vi "Read only temperature.vi"() -> ()   [LabVIEW 2013]
doc: "This example shows how to configure a measurement and take a reading."
uses:
  <vilib>/Utility/file.llb/Read From Spreadsheet File (DBL).vi
  <instrlib>/Keithley 24XX/Public/Data/Read (Single Point).vi
  <instrlib>/Keithley 24XX/Keithley 24XX.lvlib
  <vilib>/gmath/NI_Gmath.lvlib
panel:
  in  "测量间隔（毫秒）":dbl
  out "温度-时间":dbl(graph)
  out "Temperature":dbl
  in  "定标文件":string(combo)="original.txt"
  in  "Source Mode  (0: Voltage)":u16(ring) items=["Voltage", "Current"]
  in  "Compliance  Level (0.1)":dbl=0.0001
  in  "Output Level (0)":dbl=0.002
  in  "Enable Resistance Auto Range (T:Enable)":bool=TRUE
  in  "Enable Current Auto Range (T:Enable)":bool=TRUE
  in  "Enable Voltage Auto Range (T:Enable)":bool=TRUE
  in  "Resistance Manual Range (1.0)":dbl=1.0
  in  "Current Manual Range (1.0)":dbl=1.0
  in  "Voltage Manual Range (1.0)":dbl=1.0
  out "Resistance":sgl
  out "Current":sgl
  out "Voltage":sgl
  in  "Serial Configuration":T1={"Baud Rate"=9600, "Parity"=0, "Data Bits"=8, "Stop Bits"=10, "Flow Control"=0} {"Flow Control" items=["None", "XON/XOFF", "RTS/CTS", "XON/XOFF & RTS/CTS", "DTR/DSR", "XON/XOFF & DTR/DSR"]; "Stop Bits" items=["1.0"=10, "1.5"=15, "2.0"=20]; "Data Bits" items=["7"=7, "8"=8]; "Parity" items=["None", "Odd", "Even", "Mark", "Space"]; "Baud Rate" items=["300"=300, "600"=600, "1200"=1200, "2400"=2400, "4800"=4800, "9600"=9600, "19200"=19200]}
  in  "Keithley 2400\nVISA resource name":refnum<visa-resource-name>
  # "温度测量（适用于Keithley 2400） 版本：1.1"
  # "Voltage Range Settings"
  # "Current Range Settings"
  # "Resistance Range Settings"
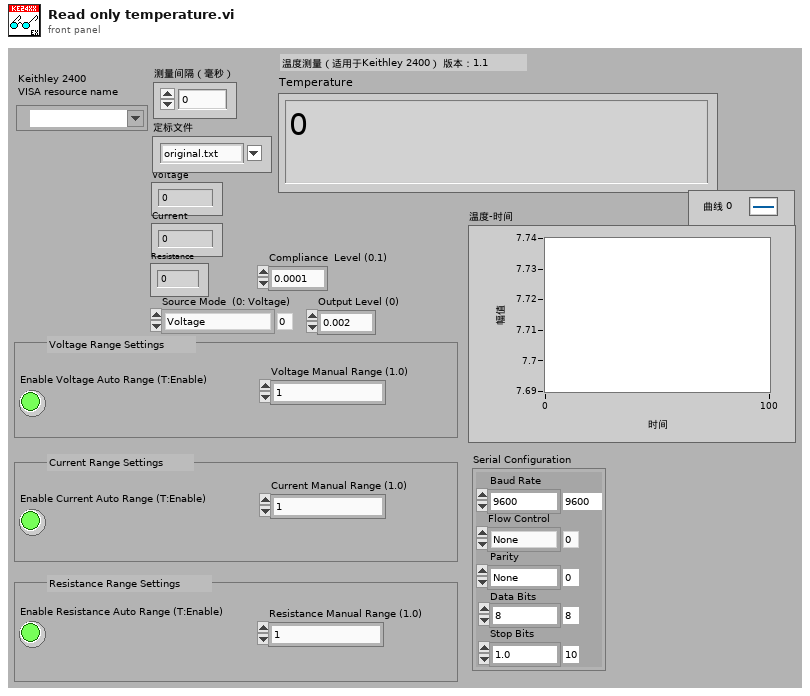
[diagram p1: front panel]
types:
  T1 = cluster{"Baud Rate":u32, "Parity":u16, "Data Bits":u16, "Stop Bits":u16, "Flow Control":u16}
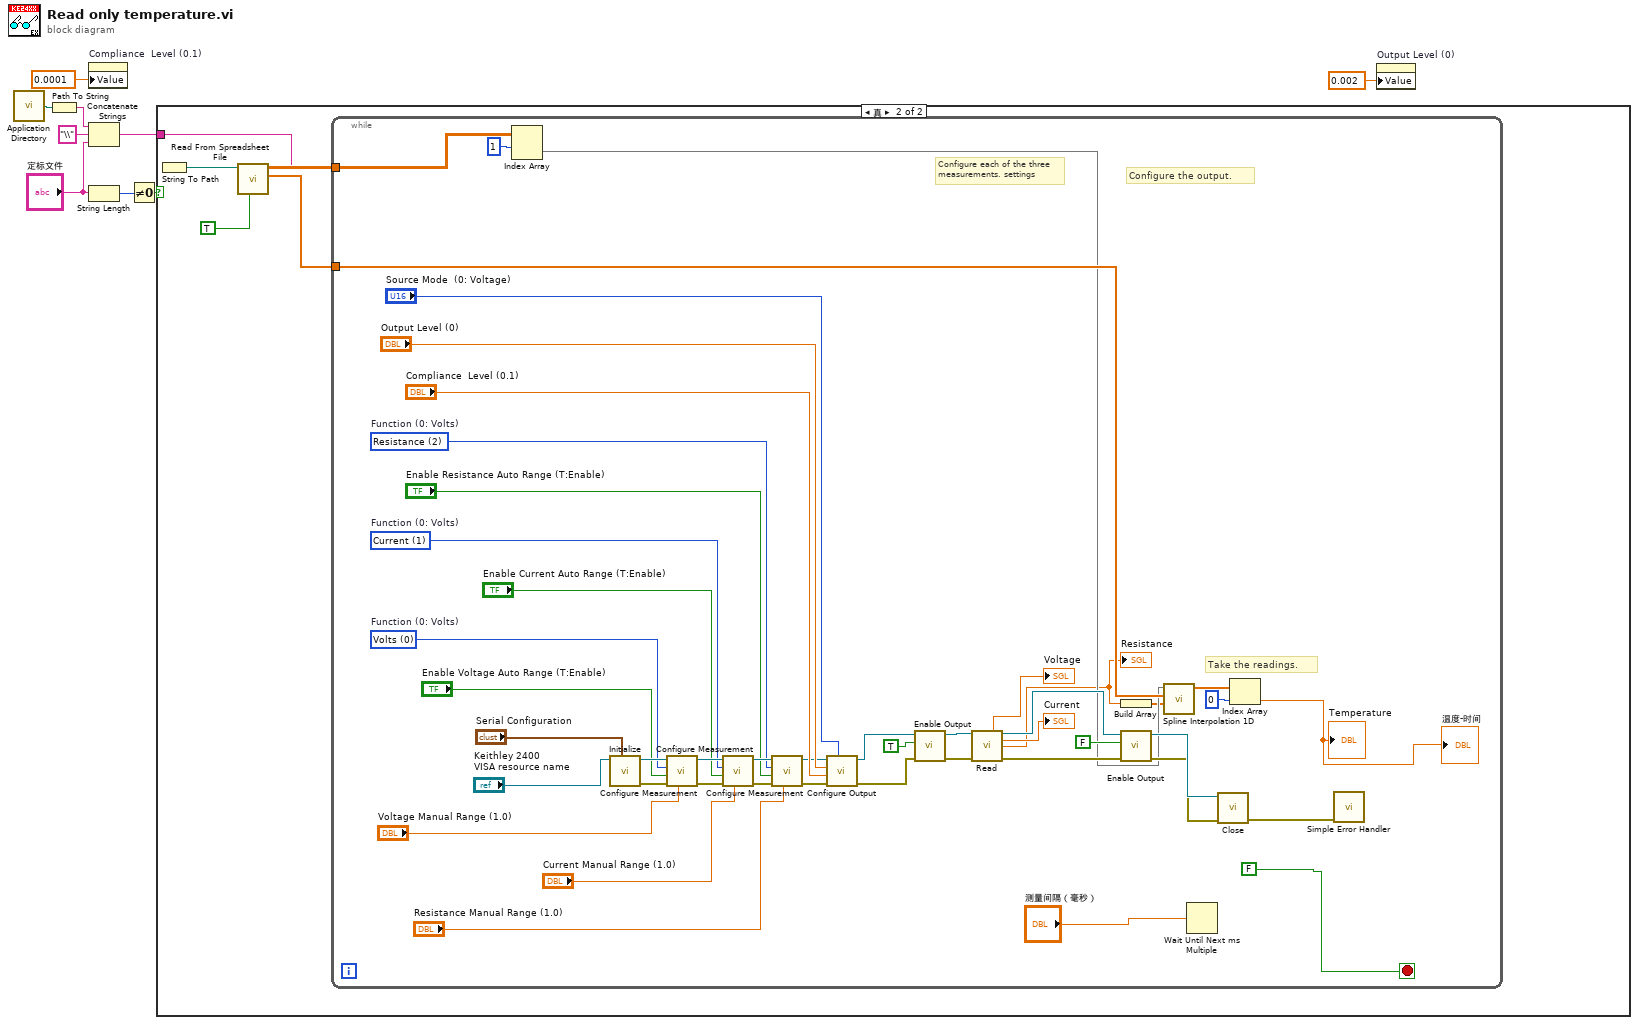
[diagram p0: block diagram]
diagram:
  n1 = call <vilib>:"Application Directory.vi"() -> ("Application Directory"=w9:path)
  n2 = Path To String(path=w9) -> (string=w8:string)
  n3 = property on="Compliance  Level (0.1)" class="DigNum (严格)"("Value"=0.0001) -> ()  [unwired: 2 in, 2 out]
  n4 = Concatenate Strings(w8, "\\", "定标文件") -> (w3:string)
  n5 = String Length(string="定标文件") -> (length=w5:i32)
  n6 = Not Equal To 0?(x=w5) -> (x != 0?=w4:bool)
  n7 = case shown="真" w4 {
    tunnel: w3 -> [_ w10]
    frame False {
    }
    frame True {
      n8 = String To Path(string=w10) -> (path=w14:path)
      n9 = call-poly <vilib>:"Read From Spreadsheet File.vi"("transpose (no:F)"=TRUE, "file path (dialog if empty)"=w14) -> ("first row"=w11:dbl[], "all rows"=w12:dbl[][])  [unwired: 5 in, 3 out]
      n10 = while {
        tunnel: w12 -> [w25]
        tunnel: w11 -> [w24]
        stop <- FALSE stop-if-true
        w47 = u16 2 items=["Volts", "Current", "Resistance"]  # Function (0: Volts)
        w48 = u16 1 items=["Volts", "Current", "Resistance"]  # Function (0: Volts)
        w49 = u16 0 items=["Volts", "Current", "Resistance"]  # Function (0: Volts)
        # "Take the readings."
        # "Configure the output."
        # "Configure each of the three measurements. settings"
        n11 = Index Array(array=w25, index (row)=1) -> (element=w23:dbl[])  [unwired: 1 in]
        n12 = call <instrlib>:"Initialize.vi"("Serial Configuration"="Serial Configuration", "VISA resource name"="Keithley 2400\nVISA resource name") -> ("error out"=w54:errorcluster, "VISA resource name out"=w55:refnum<visa-resource-name>)  [unwired: 8 in]
        n13 = call <instrlib>:"Configure Measurement.vi"("Manual Range (1.0)"="Voltage Manual Range (1.0)", "error in (no error)"=w54, "Enable Auto Range (T:Enable)"="Enable Voltage Auto Range (T:Enable)", "Function (0: Volts)"=w49, "VISA resource name"=w55) -> ("error out"=w52:errorcluster, "VISA resource name out"=w53:refnum<visa-resource-name>)  [unwired: 5 in]
        n14 = call <instrlib>:"Configure Measurement.vi"("Manual Range (1.0)"="Current Manual Range (1.0)", "error in (no error)"=w52, "Enable Auto Range (T:Enable)"="Enable Current Auto Range (T:Enable)", "Function (0: Volts)"=w48, "VISA resource name"=w53) -> ("error out"=w51:errorcluster, "VISA resource name out"=w50:refnum<visa-resource-name>)  [unwired: 5 in]
        n15 = call <instrlib>:"Configure Measurement.vi"("Manual Range (1.0)"="Resistance Manual Range (1.0)", "error in (no error)"=w51, "Enable Auto Range (T:Enable)"="Enable Resistance Auto Range (T:Enable)", "Function (0: Volts)"=w47, "VISA resource name"=w50) -> ("error out"=w28:errorcluster, "VISA resource name out"=w27:refnum<visa-resource-name>)  [unwired: 5 in]
        n16 = call <instrlib>:"Configure Output.vi"("Source Mode  (0: Voltage)"="Source Mode  (0: Voltage)", "error in (no error)"=w28, "Compliance  Level (0.1)"="Compliance  Level (0.1)", "Output Level (0)"="Output Level (0)", "VISA resource name"=w27) -> ("error out"=w30:errorcluster, "VISA resource name out"=w31:refnum<visa-resource-name>)  [unwired: 5 in]
        n17 = call <instrlib>:"Enable Output.vi"("error in (no error)"=w30, "Enable Output (T: Enable)"=TRUE, "VISA resource name"=w31) -> ("error out"=w33:errorcluster, "VISA resource name out"=w32:refnum<visa-resource-name>)  [unwired: 7 in]
        n18 = call-poly <instrlib>:"Read.vi"("VISA resource name"=w32, "error in (no error)"=w33) -> ("Voltage"=→"Voltage":sgl, "VISA resource name out"=w34:refnum<visa-resource-name>, "Current"=→"Current":sgl, "Resistance"=w22:sgl, "error out"=w35:errorcluster)  [unwired: 7 in, 2 out]
        "Resistance" <- w22
        n19 = Build Array(w22) -> (w21:sgl[])
        n20 = call <instrlib>:"Enable Output.vi"("error in (no error)"=w35, "Enable Output (T: Enable)"=FALSE, "VISA resource name"=w34) -> ("error out"=w36:errorcluster, "VISA resource name out"=w37:refnum<visa-resource-name>)  [unwired: 7 in]
        n21 = call <vilib>:"Spline Interpolation 1D.vi"("xi"=w21, "X"=w24, "Y"=w23) -> ("yi"=w20:dbl[])  [unwired: 6 in, 2 out]
        n22 = Wait Until Next ms Multiple(millisecond multiple="测量间隔（毫秒）") -> ()  [unwired: 1 out]
        n23 = call <instrlib>:"Close.vi"("error in (no error)"=w36, "VISA resource name"=w37) -> ("error out"=w60:errorcluster)  [unwired: 9 in]
        n24 = Index Array(array=w20, index=0) -> (element=→"Temperature" →"温度-时间":dbl)
        n25 = call <vilib>:"Simple Error Handler.vi"("error in (no error)"=w60) -> ()  [unwired: 4 in, 5 out]
      }
    }
  }
  n26 = property on="Output Level (0)" class="DigNum (严格)"("Value"=0.002) -> ()  [unwired: 2 in, 2 out]
